vi "getPostProcessing.vi"() -> ()   [LabVIEW 2013]
uses:
  Globals/measurementGlobal.vi
panel:
  out "output array 2":dbl[][](array[numeric])
  out "output array":dbl[][](array[numeric])
  out "appended array":dbl[](array[numeric])
  out "Analogue Data (volts)":dbl[][](array[numeric])
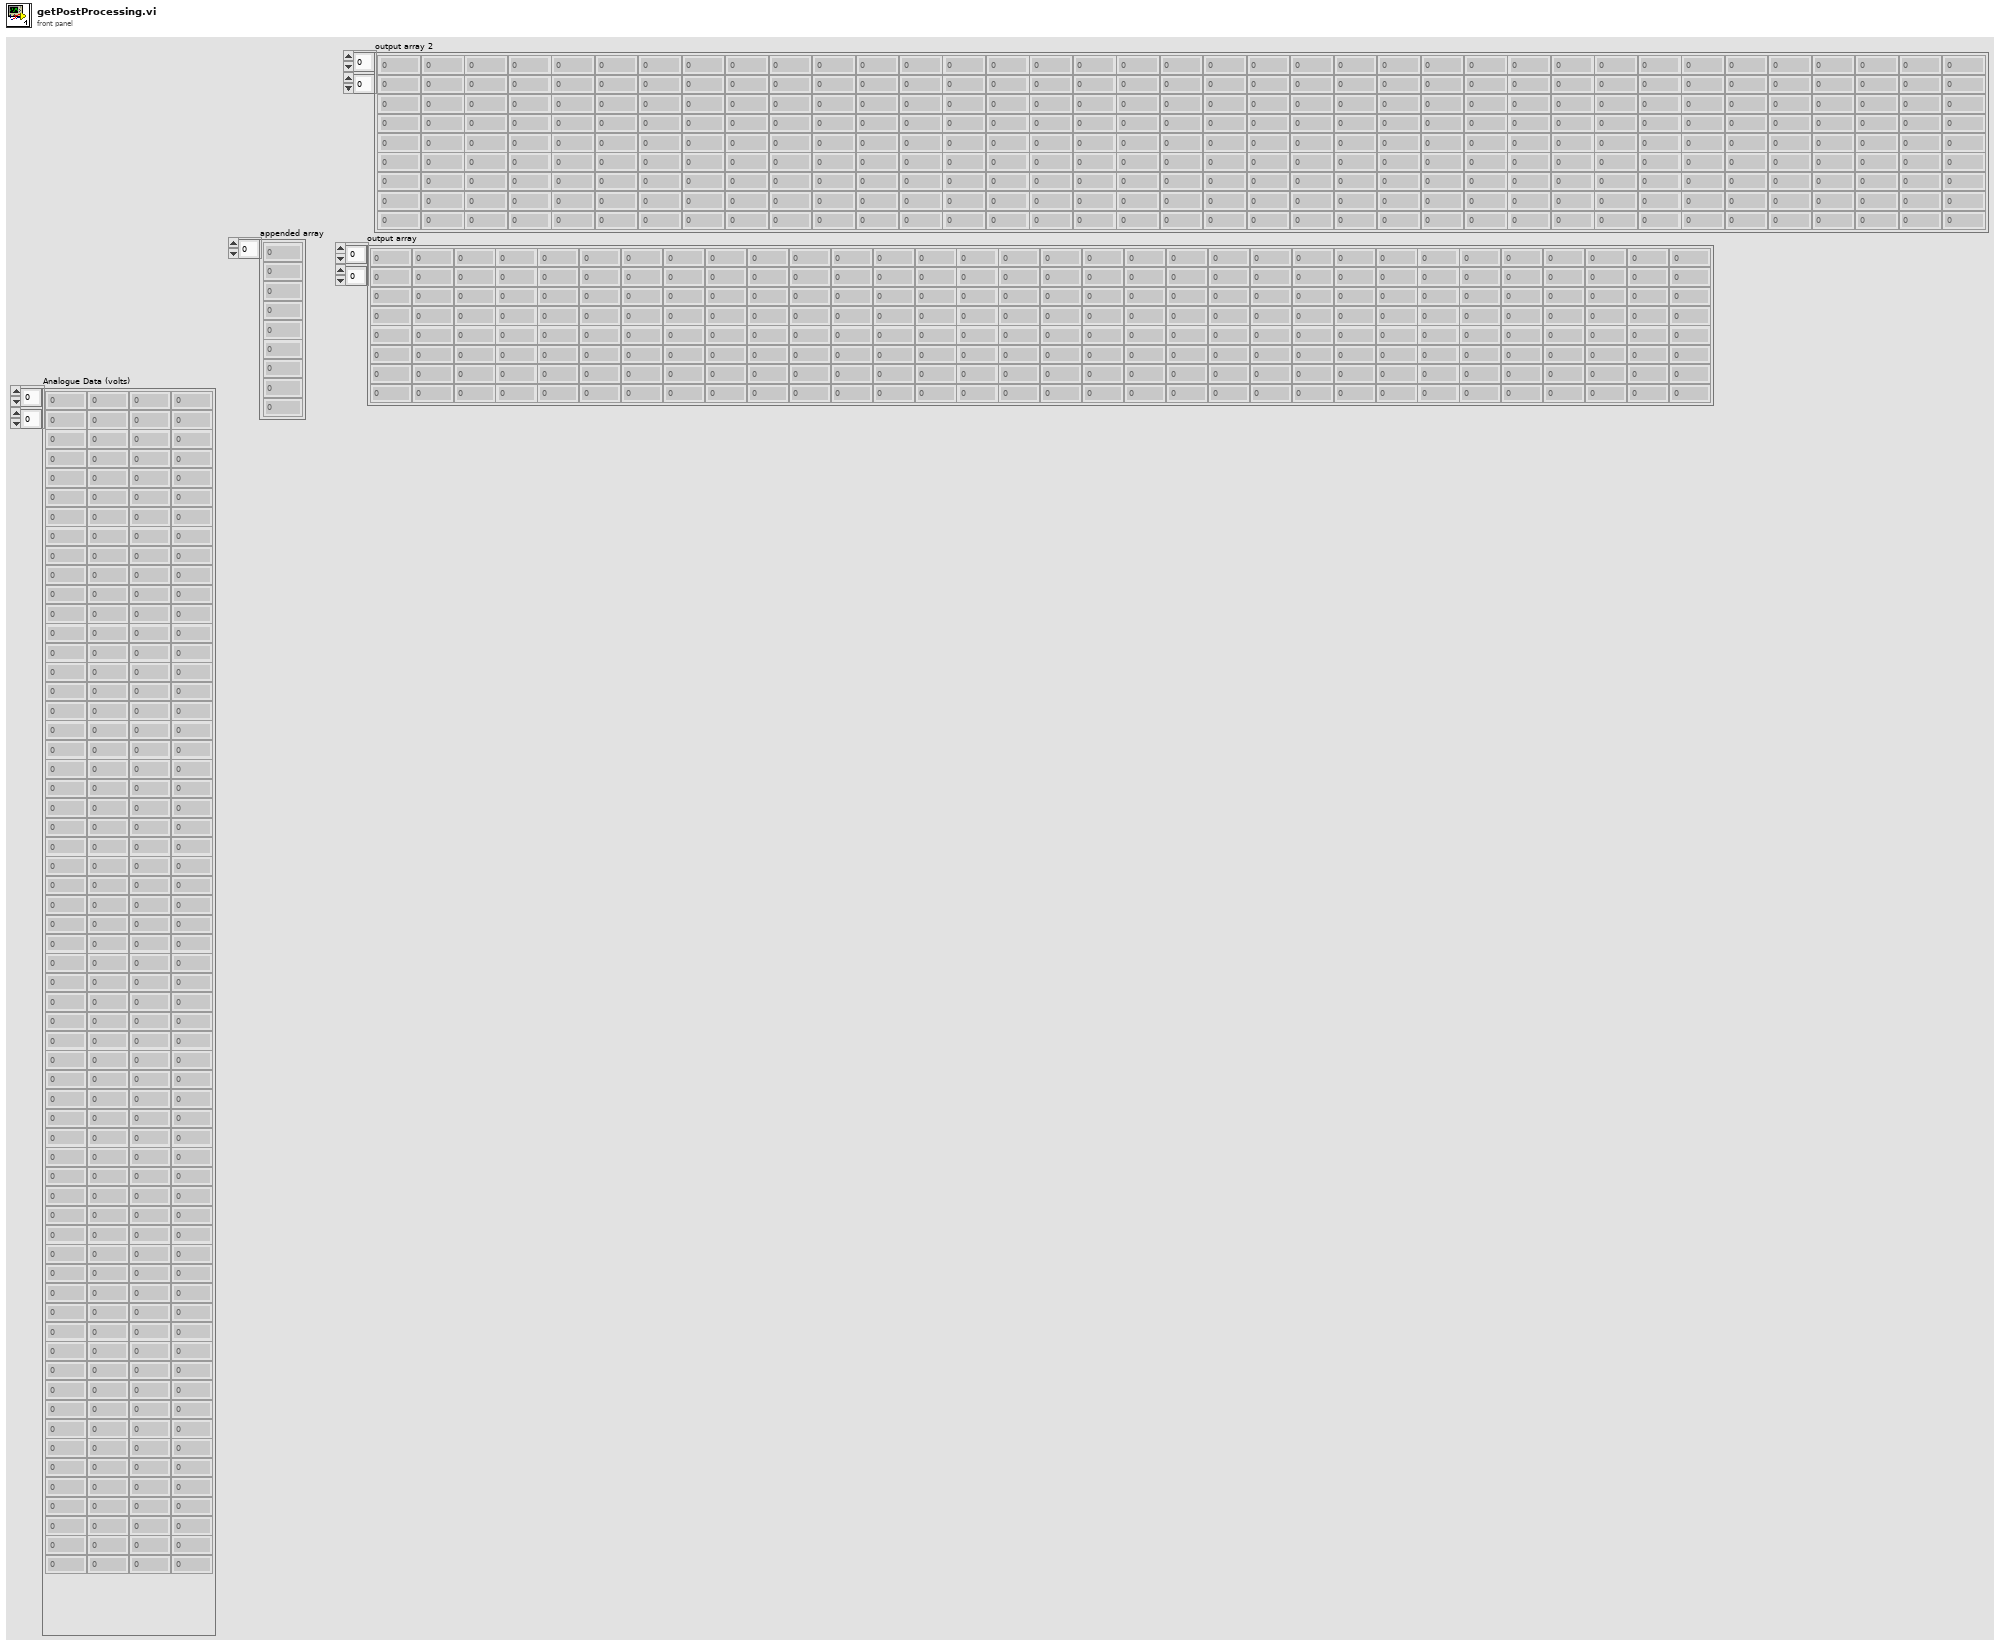
[diagram p1: front panel]
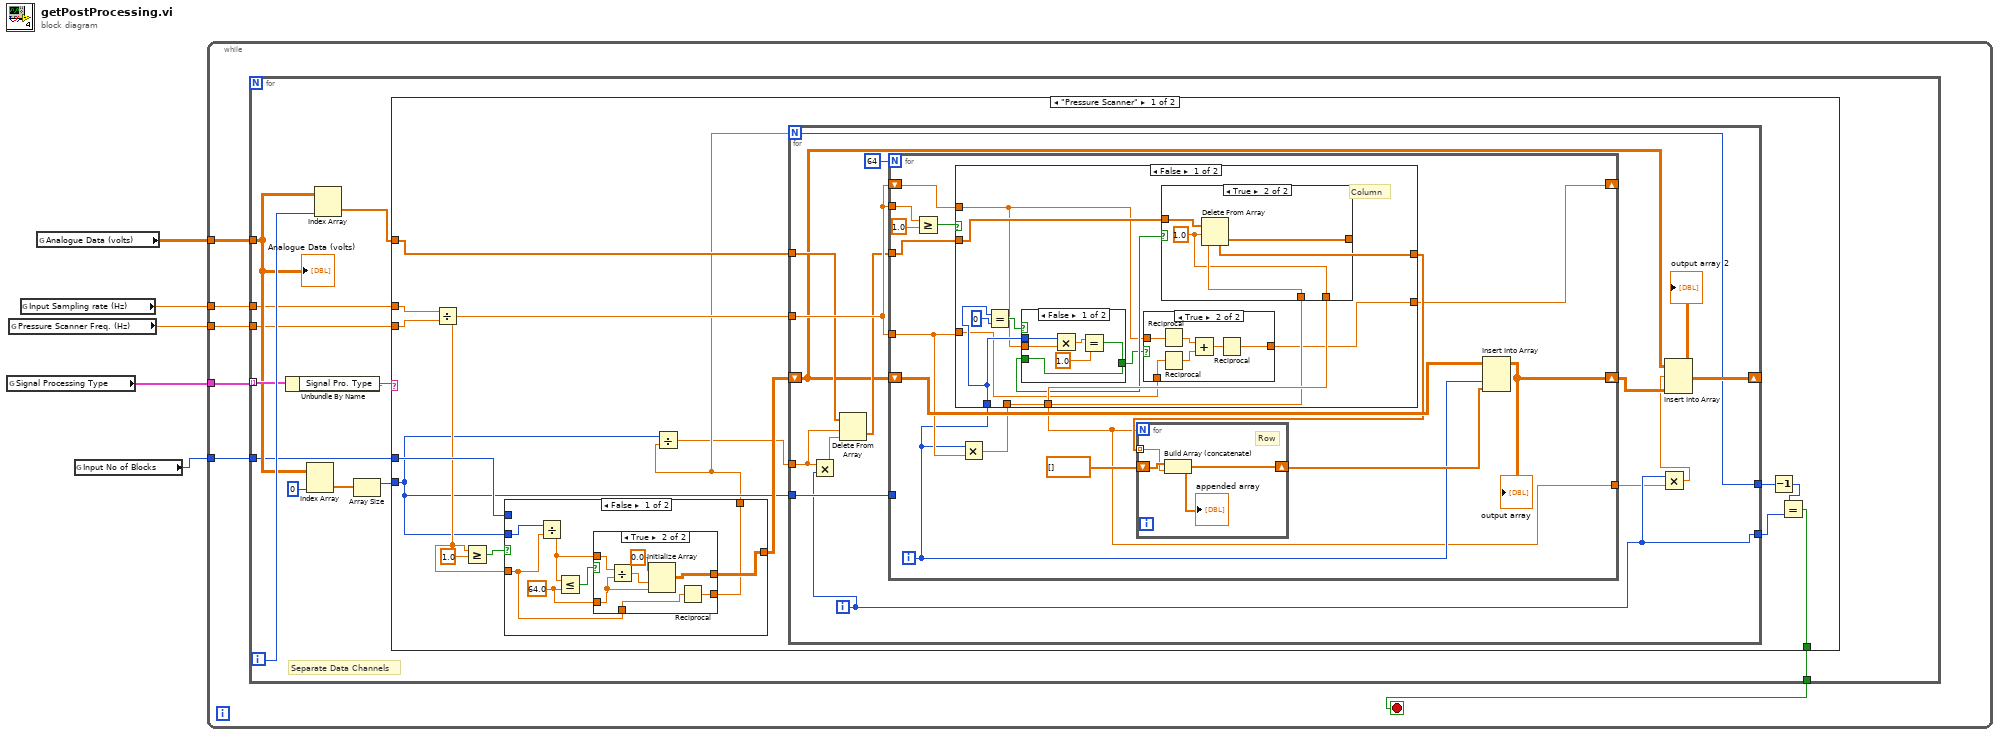
[diagram p0: block diagram]
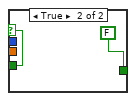
[diagram p3: hidden frame]
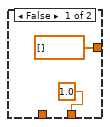
[diagram p4: hidden frame]
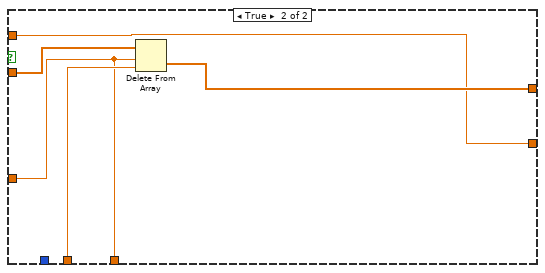
[diagram p5: hidden frame]
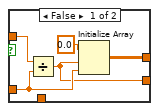
[diagram p6: hidden frame]
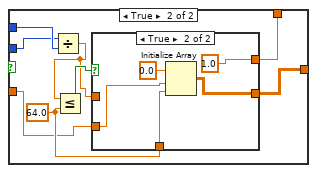
[diagram p7: hidden frame]
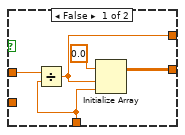
[diagram p8: hidden frame]
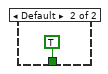
[diagram p9: hidden frame]
diagram:
  n1 = global read "measurementGlobal.vi" "Signal Processing Type"() -> (w5:cluster{"Signal Pro. Type":string}[])
  n2 = global read "measurementGlobal.vi" "Pressure Scanner Freq. (Hz)"() -> (w2:dbl)
  n3 = global read "measurementGlobal.vi" "Input Sampling rate (Hz)"() -> (w3:dbl)
  n4 = global read "measurementGlobal.vi" "Analogue Data (volts)"() -> (w4:dbl[][])
  n5 = global read "measurementGlobal.vi" "Input No of Blocks"() -> (w1:i32)
  n6 = while {
    tunnel: w5 -> [w11]
    tunnel: w4 -> [w10]
    tunnel: w3 -> [w9]
    tunnel: w2 -> [w8]
    tunnel: w1 -> [w7]
    stop <- w6 stop-if-true
    n7 = for {
      tunnel: w11 -> [w20] mode=indexing
      tunnel: w10 -> [w19]
      tunnel: w9 -> [w15]
      tunnel: w8 -> [w14]
      tunnel: w7 -> [w13]
      tunnel: [w12] -> w6
      i -> [w22]
      # "Separate Data Channels"
      n8 = Unbundle By Name(w20) -> ("Signal Pro. Type"=w23:string)
      n9 = Index Array(array=w19, index (col)=0 ("disabled index (col)")) -> (element=w17:dbl[])  [unwired: 1 in]
      n10 = Index Array(array=w19, index (col)=w22) -> (element=w21:dbl[])  [unwired: 1 in]
      n11 = Array Size(array=w17) -> (size(s)=w16:i32)
      n12 = case shown="\"Pressure Scanner\"" w23 {
        tunnel: w21 -> [w36 _]
        tunnel: w14 -> [w38 _]
        tunnel: w15 -> [w37 _]
        tunnel: w16 -> [w26 _]
        tunnel: w13 -> [w33 _]
        tunnel: [w27 TRUE] -> w12
        frame "Pressure Scanner" {
          n13 = Divide(x=w37, y=w38) -> (x/y=w32:dbl)
          n14 = Greater Or Equal?(x=w32, y=1.0) -> (x >= y?=w34:bool)
          n15 = case shown="False" w34 {
            tunnel: w33 -> [_ w134]
            tunnel: w26 -> [w114 w133]
            tunnel: w32 -> [w108 w128]
            tunnel: [w110 w130] -> w31
            tunnel: [w109 w129] -> w25
            frame False {
              w112 = 64.0 ("y")
              n16 = Divide(x=w114, y=w108) -> (x/y=w111:dbl)
              n17 = Less Or Equal?(x=w111, y=w112) -> (x <= y?=w113:bool)
              n18 = case shown="True" w113 {
                tunnel: w112 -> [w117 w122]
                tunnel: w111 -> [w118 w123]
                tunnel: [w116 w120] -> w110
                tunnel: [w115 w124] -> w109
                tunnel: w108 -> [_ w125]
                frame False {
                  n19 = Divide(x=w118, y=w117) -> (x/y=w115:dbl)
                  n20 = Initialize Array(0.0 ("element"), w115, w117) -> (w116:dbl[][])
                }
                frame True {
                  n21 = Divide(x=w123, y=w122) -> (x/y=w121:dbl)
                  n22 = Initialize Array(0.0 ("element"), w121, w122) -> (w120:dbl[][])
                  n23 = Reciprocal(x=w125) -> (1/x=w124:dbl)
                }
              }
            }
            frame True {
              w131 = 64.0 ("y")
              n24 = Divide(x=w133, y=w134) -> (x/y=w127:dbl)
              n25 = Less Or Equal?(x=w127, y=w131) -> (x <= y?=w132:bool)
              n26 = case shown="True" w132 {
                tunnel: w131 -> [w135 w143]
                tunnel: [w137 w142] -> w130
                tunnel: w127 -> [w138 _]
                tunnel: [w136 1.0] -> w129
                tunnel: w128 -> [_ w140]
                frame False {
                  n27 = Divide(x=w138, y=w135) -> (x/y=w136:dbl)
                  n28 = Initialize Array(0.0 ("element"), w136, w135) -> (w137:dbl[][])
                }
                frame True {
                  n29 = Initialize Array(0.0 ("element"), w140, w143) -> (w142:dbl[][])
                }
              }
            }
          }
          n30 = Divide(x=w26, y=w25) -> (x/y=w24:dbl)
          n31 = for {
            N: w25 -> [w45]
            tunnel: w36 -> [w48]
            tunnel: w26 -> [w52]
            tunnel: w32 -> [w51]
            shift-right: [w49] -> _
            shift-left: w31 -> [w43]
            tunnel: [w42] -> w28
            tunnel: [w45] -> w30
            tunnel: w24 -> [w44]
            i -> [w42]
            n32 = Multiply(x=w44, y=w42) -> (x*y=w46:dbl)
            n33 = Delete From Array(array=w48, length=w44, index=w46) -> (deleted portion=w47:dbl[])  [unwired: 1 out]
            n34 = for {
              N: 64 -> [_]
              tunnel: w52 -> [_]
              tunnel: w47 -> [w65]
              tunnel: w51 -> [w62]
              shift-right: [w60] -> w50
              shift-left: w43 -> [w67]
              tunnel: w51 -> [w57]
              shift-right: [w54] -> _
              shift-left: w51 -> [w55]
              tunnel: [w53] -> w40
              i -> [w59]
              n35 = Greater Or Equal?(x=w57, y=1.0) -> (x >= y?=w56:bool)
              n36 = Multiply(x=w59, y=w62) -> (x*y=w63:dbl)
              n37 = case shown="False" w56 {
                tunnel: w65 -> [w79 w104]
                tunnel: [w78 w103] -> w64
                tunnel: w63 -> [w76 w102]
                tunnel: w62 -> [w68 w101]
                tunnel: w59 -> [w72 _]
                tunnel: [w77 w101] -> w53
                tunnel: w55 -> [w71 w100]
                tunnel: [w69 w100] -> w54
                frame False {
                  # "Column"
                  n38 = Equal?(x=w72, y=0) -> (x = y?=w74:bool)
                  n39 = case shown="False" w74 {
                    selector: w74 -> [_ w93]
                    tunnel: [w87 w93] -> w73
                    tunnel: w72 -> [w91 _]
                    tunnel: w71 -> [w90 _]
                    tunnel: [w87 FALSE] -> w70
                    frame False {
                      n40 = Multiply(x=w91, y=w90) -> (x*y=w89:dbl)
                      n41 = Equal?(x=w89, y=1.0) -> (x = y?=w87:bool)
                    }
                    frame True {
                    }
                  }
                  n42 = case shown="True" w70 {
                    tunnel: w71 -> [w80 w86]
                    tunnel: [w80 w81] -> w69
                    tunnel: w68 -> [_ w85]
                    frame False {
                    }
                    frame True {
                      n43 = Reciprocal(x=w86) -> (1/x=w84:dbl)
                      n44 = Reciprocal(x=w85) -> (1/x=w83:dbl)
                      n45 = Add(x=w84, y=w83) -> (x+y=w82:dbl)
                      n46 = Reciprocal(x=w82) -> (1/x=w81:dbl)
                    }
                  }
                  n47 = case shown="True" w73 {
                    tunnel: w79 -> [_ w99]
                    tunnel: w76 -> [_ w98]
                    tunnel: [dbl[] [] ("Analogue Data (volts)") w97] -> w78
                    tunnel: [1.0 ("y") w96] -> w77
                    frame False {
                    }
                    frame True {
                      w96 = 1.0 ("y")
                      n48 = Delete From Array(array=w99, length=w96, index=w98) -> (deleted portion=w97:dbl[])  [unwired: 1 out]
                    }
                  }
                }
                frame True {
                  n49 = Delete From Array(array=w104, length=w101, index=w102) -> (deleted portion=w103:dbl[])  [unwired: 1 out]
                }
              }
              n50 = for {
                N: w53 -> [_]
                shift-right: [w106] -> w66
                shift-left: dbl[] [] -> [w107]
                tunnel: w64 -> [w105] mode=indexing
                # "Row"
                n51 = Build Array (concatenate)(w107, w105) -> (w106:dbl[])
                "appended array" <- w106
              }
              n52 = Insert Into Array(array=w67, index (col)=w59, new element=w66) -> (w60:dbl[][])  [unwired: 1 in]
              "output array" <- w60
            }
            n53 = Multiply(x=w42, y=w40) -> (x*y=w41:dbl)
            n54 = Insert Into Array(array=w43, index (row)=w41, new element=w50) -> (w49:dbl[][])  [unwired: 1 in]
            "output array 2" <- w49
          }
          n55 = Decrement(x=w30) -> (x-1=w29:i32)
          n56 = Equal?(x=w29, y=w28) -> (x = y?=w27:bool)
        }
        frame Default {
        }
      }
      "Analogue Data (volts)" <- w19
    }
  }
